vi "Configure User Domain Range.vi"(6 "Range Stop (2E+9 Hz)":dbl=2000000000.0, 7 "Range Start (1E+9 Hz)":dbl=1000000000.0, 8 "error in (no error)":errorcluster, 9 "User Domain (1)":dbl=1.0, 10 "Channel (1)":i32=1, 11 "VISA resource name":refnum<visa-resource-name>) -> (0 "error out":errorcluster, 3 "VISA resource name out":refnum<visa-resource-name>)   [LabVIEW 2018, in "Keysight PNA Series.lvlib"]
doc: "Configure User Domain Range."
uses:
  Keysight PNA Series.lvlib
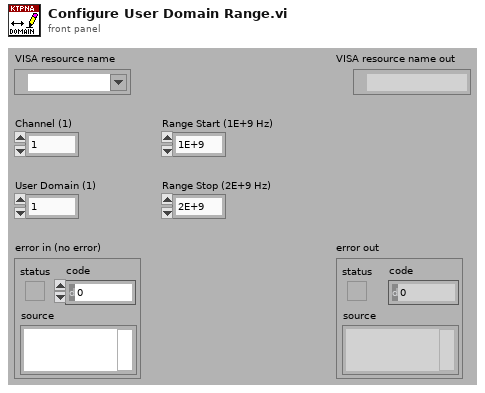
[diagram p1: front panel]
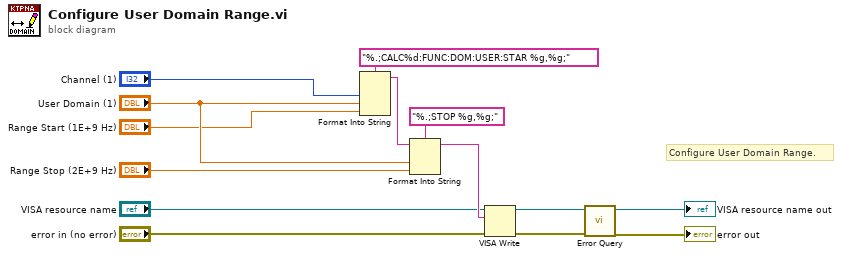
[diagram p0: block diagram]
diagram:
  # "Configure User Domain Range."
  n1 = Format Into String(format string="%.;CALC%d:FUNC:DOM:USER:STAR %g,%g;", "Channel (1)", "User Domain (1)", "Range Start (1E+9 Hz)") -> (resulting string=w11:string)  [unwired: 2 in, 1 out]
  n2 = Format Into String(format string="%.;STOP %g,%g;", initial string=w11, "User Domain (1)", "Range Stop (2E+9 Hz)") -> (resulting string=w8:string)  [unwired: 1 in, 1 out]
  n3 = VISA Write(VISA resource name="VISA resource name", write buffer=w8, error in (no error)="error in (no error)") -> (VISA resource name out=w5:refnum<visa-resource-name>, error out=w4:errorcluster)  [unwired: 1 out]
  n4 = call "Error Query.vi"("error in (no error)"=w4, "VISA resource name"=w5) -> ("error out"=→"error out":errorcluster, "VISA resource name out"=→"VISA resource name out":refnum<visa-resource-name>)  [unwired: 6 in, 2 out]
